vi "Triax320 SetPosition.vi"(7 "Grating":u8(ring) items=["1", "2", "3"], 8 "error in (no error)":errorcluster, 9 "Refnum Cmde":refnum<vi>, 10 "Lambda":dbl=100.0 caption="Longueur d'ondes(nm)" format="%#.4g", 11 "Triax VISA Rsrc":refnum<visa-resource-name>="SR530") -> (0 "error out":errorcluster, 1 "Step Out":u32=100 caption="Longueur d'ondes(Steps)", 2 "Lambda Out":dbl=100.0 caption="Longueur d'ondes(nm)", 3 "Triax VISA Rsrc Out":refnum<visa-resource-name>="SR530")   [LabVIEW 2019]
uses:
  <userlib>/Triax320/TriaxParams.ctl
panel:
  out "Moving":bool
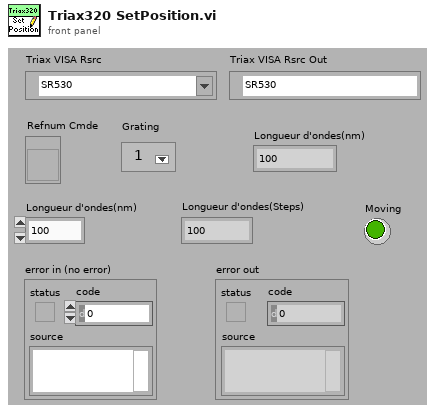
[diagram p1: front panel]
types:
  T1 = enum16{"Error", "Read Postion", "Set Position", "Wait Done"}
  T2 = typedef "TriaxParams.ctl" = enum16{"Grating", "CalOffset", "Line Density (grv/mm)", "Input Slit (mm)", "Output Slit (mm)", "Both Slit (mm)", "Grating Desc.", "Wavelenght Correction", "Tous"}
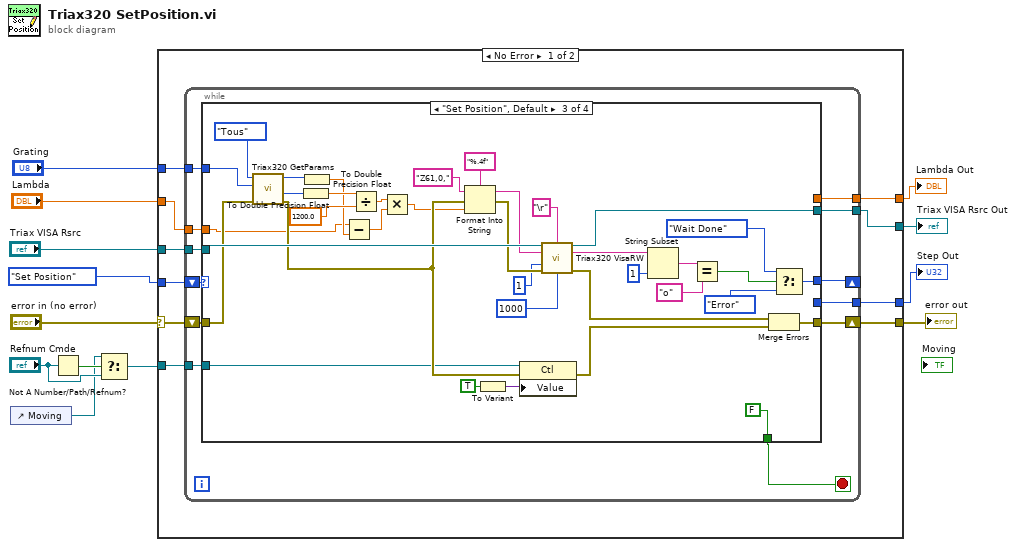
[diagram p0: block diagram]
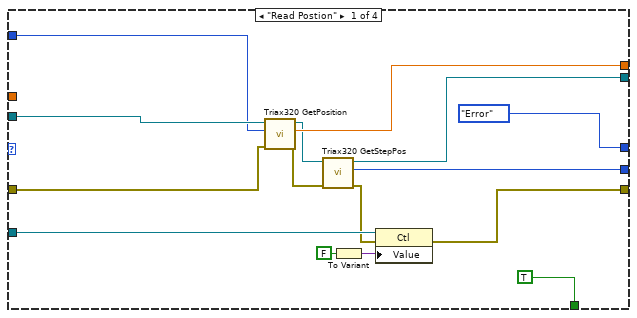
[diagram p2: hidden frame]
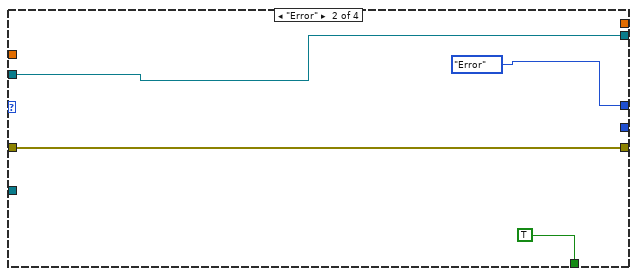
[diagram p3: hidden frame]
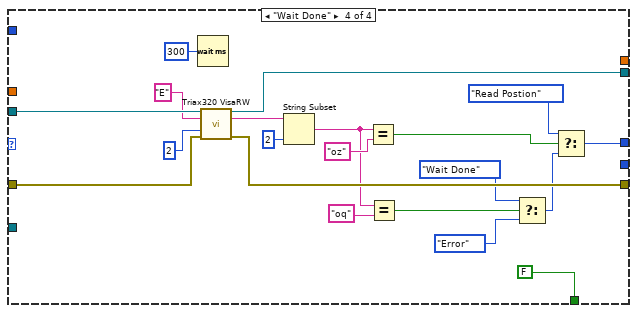
[diagram p4: hidden frame]
diagram:
  n1 = control-ref of="Moving"() -> (w2:refnum<vi>)
  n2 = Not A Number/Path/Refnum?(number/path/refnum="Refnum Cmde") -> (NaN/Path/Refnum?=w5:bool)
  n3 = Select(t=w2, s=w5, f="Refnum Cmde") -> (s? t:f=w3:refnum<vi>)
  n4 = case shown="No Error" "error in (no error)" {
    selector: "error in (no error)" -> [w22 w112]
    tunnel: "Triax VISA Rsrc" -> [w23 w113]
    tunnel: "Lambda" -> [w21 _]
    tunnel: [w20 _] -> w10
    tunnel: [w19 w112] -> w9
    tunnel: [w18 w113] -> w8
    tunnel: T1."Set Position" -> [w17 _]
    tunnel: "Grating" -> [w16 _]
    tunnel: w3 -> [w15 _]
    tunnel: [w14 _] -> w1
    frame No Error {
      n5 = while {
        shift-right: [w33] -> _
        shift-left: w17 -> [w35]
        tunnel: w23 -> [w32]
        shift-right: [w30] -> w19
        shift-left: w22 -> [w31]
        tunnel: [w29] -> w18
        tunnel: w21 -> [w26]
        tunnel: [w28] -> w20
        tunnel: w15 -> [w27]
        tunnel: w16 -> [w25]
        tunnel: [w24] -> w14
        stop <- w34 stop-if-true
        n6 = case shown="\"Set Position\", Default" w35 {
          tunnel: [TRUE TRUE FALSE FALSE] -> w34
          tunnel: [T1."Error" T1."Error" w82 w103] -> w33
          tunnel: w32 -> [w49 w52 w90 w110]
          tunnel: w31 -> [w48 w53 w68 w100]
          tunnel: [w43 w53 w72 w109] -> w30
          tunnel: [w37 w52 w88 w108] -> w29
          tunnel: w26 -> [_ _ w57 _]
          tunnel: [w47 _ _ _] -> w28
          tunnel: w27 -> [w42 _ w61 _]
          tunnel: w25 -> [w41 _ w69 _]
          tunnel: [w36 _ _ _] -> w24
          frame "Read Postion" {
            n7 = call <userlib>:"Triax320 GetPosition.vi"("error in (no error)"=w48, "Grating"=w41, "Triax VISA Rsrc"=w49) -> ("error out"=w39:errorcluster, "Lambda Out"=w47:dbl, "Triax VISA Rsrc Out"=w40:refnum<visa-resource-name>)  [unwired: 6 in]
            n8 = call <userlib>:"Triax320 GetStepPos.vi"("error in (no error)"=w39, "Triax VISA Rsrc"=w40) -> ("error out"=w38:errorcluster, "Step Out"=w36:u32, "Triax VISA Rsrc Out"=w37:refnum<visa-resource-name>)  [unwired: 7 in]
            n9 = To Variant(anything=FALSE) -> (Variant=w45:variant)
            n10 = property class="Ctl"(reference=w42, error in=w38, "Value"=w45) -> (error out=w43:errorcluster)  [unwired: 1 out]
          }
          frame "Error" {
          }
          frame "Set Position", Default {
            n11 = call <userlib>:"Triax320 GetParams.vi"("error in"=w68, "Grating"=w69, "Param"=TriaxParams."Tous") -> ("error out"=w67:errorcluster, "LineDensity"=w60:u32, "WvlCorr"=w59:i32)  [unwired: 2 in, 4 out]
            n12 = To Double Precision Float(number=w60) -> (double precision float=w66:dbl)
            n13 = To Double Precision Float(number=w59) -> (double precision float=w58:dbl)
            n14 = Subtract(x=w57, y=w58) -> (x-y=w56:dbl)
            n15 = Divide(x=w66, y=1200.0) -> (x/y=w64:dbl)
            n16 = Multiply(x=w64, y=w56) -> (x*y=w55:dbl)
            n17 = Format Into String(format string="%.4f" ("chaîne"), initial string="Z61,0," ("chaîne"), error in=w67, w55) -> (resulting string=w79:string, error out=w78:errorcluster)
            n18 = To Variant(anything=TRUE) -> (Variant=w62:variant)
            n19 = property class="Ctl"(reference=w61, error in=w67, "Value"=w62) -> (error out=w71:errorcluster)  [unwired: 1 out]
            n20 = call <userlib>:"Triax320 VisaRW.vi"("VISA Rsrc"=w90, "EOS (Aucun)"="\r" ("chaîne"), "ChaineCom"=w79, "Nbcaract"=u32 1, "error in (no error)"=w78, "Timeout ms"=u32 1000) -> ("VISA Rsrc Out"=w88:refnum<visa-resource-name>, "ChaineRep"=w87:string, "error out"=w89:errorcluster)  [unwired: 4 in, 3 out]
            n21 = String Subset(string=w87, length (rest)=1 ("longueur (reste)")) -> (substring=w84:string)  [unwired: 1 in]
            n22 = Equal?(x=w84, y="o") -> (x = y?=w83:bool)
            n23 = Merge Errors(w89, w71) -> (w72:errorcluster)
            n24 = Select(t=T1."Wait Done", s=w83, f=T1."Error") -> (s? t:f=w82:T1)
          }
          frame "Wait Done" {
            n25 = Wait (ms)(milliseconds to wait=u32 300 ("attente (ms)")) -> ()  [unwired: 1 out]
            n26 = call <userlib>:"Triax320 VisaRW.vi"("VISA Rsrc"=w110, "ChaineCom"="E" ("chaîne"), "Nbcaract"=u32 2, "error in (no error)"=w100) -> ("VISA Rsrc Out"=w108:refnum<visa-resource-name>, "ChaineRep"=w107:string, "error out"=w109:errorcluster)  [unwired: 6 in, 3 out]
            n27 = String Subset(string=w107, length (rest)=2 ("longueur (reste)")) -> (substring=w97:string)  [unwired: 1 in]
            n28 = Equal?(x=w97, y="oz") -> (x = y?=w104:bool)
            n29 = Equal?(x=w97, y="oq") -> (x = y?=w95:bool)
            n30 = Select(t=T1."Wait Done", s=w95, f=T1."Error") -> (s? t:f=w94:T1)
            n31 = Select(t=T1."Read Postion", s=w104, f=w94) -> (s? t:f=w103:T1)
          }
        }
      }
    }
    frame Error {
    }
  }
  "error out" <- w9
  "Lambda Out" <- w10
  "Triax VISA Rsrc Out" <- w8
  "Step Out" <- w1
